vi "convert--chessboard_index to chess_square (string).vi"(1 "chessboard_index":T1) -> (0 "chess square (string)":string)   [LabVIEW 2020, in "core.lvlib"]
uses:
  core.lvlib
  core_data/chessboard_index.ctl
  core_data/core_data.lvlib
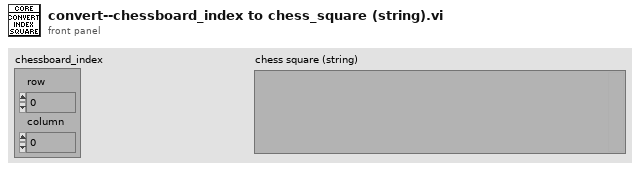
[diagram p1: front panel]
types:
  T1 = typedef "core.lvlib/core_data.lvlib/chessboard_index.ctl" = cluster{"row":u8, "column":u8}
  T2 = typedef "core.lvlib/core_data.lvlib/chess_square--chess notation.ctl" = cluster{"file":T3, "rank":T4}
  T3 = typedef "core.lvlib/core_data.lvlib/file--enum.ctl" = enum16{"a", "b", "c", "d", "e", "f", "g", "h"}
  T4 = typedef "core.lvlib/core_data.lvlib/rank--enum.ctl" = enum16{"1", "2", "3", "4", "5", "6", "7", "8"}
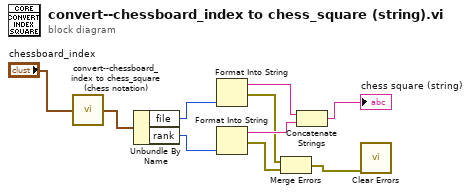
[diagram p0: block diagram]
diagram:
  n1 = call "convert--chessboard_index to chess_square (chess notation).vi"("chessboard_index"="chessboard_index") -> ("chess_square (chess notation)"=w9:T2)
  n2 = Unbundle By Name(w9) -> ("file"=w8:T3, "rank"=w5:T4)
  n3 = Format Into String(w8) -> (resulting string=w7:string, error out=w3:errorcluster)  [unwired: 3 in]
  n4 = Format Into String(w5) -> (resulting string=w6:string, error out=w2:errorcluster)  [unwired: 3 in]
  n5 = Merge Errors(w3, w2) -> (w1:errorcluster)
  n6 = Concatenate Strings(w7, w6) -> (→"chess square (string)":string)
  n7 = call <vilib>:"Clear Errors.vi"("error in (no error)"=w1) -> ()  [unwired: 5 in, 2 out]
